vi "get raw data.vi"(8 "error in (no error)":errorcluster, 11 "Task.lvclass in":refnum<class "Task.lvclass">) -> (0 "error out":errorcluster, 2 "data":T1, 3 "Task.lvclass out":refnum<class "Task.lvclass">)   [LabVIEW 2020, in "Tasks.lvlib" / "Task.lvclass"]
uses:
  Task.lvclass
  data.ctl
  SignalConversion/DAQChannelRawData.ctl
  Task.lvclass/Task.ctl
  SignalConversion/SignalConverson.lvlib
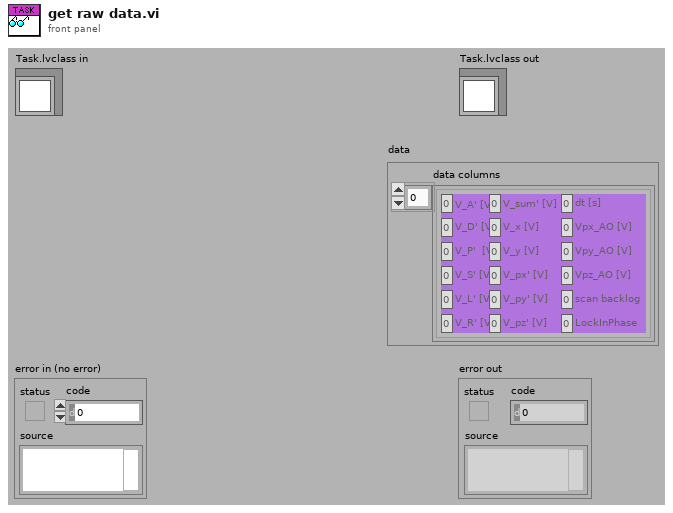
[diagram p1: front panel]
types:
  T1 = typedef "Tasks.lvlib/Task.lvclass/data.ctl" = cluster{"data columns":T2[]}
  T2 = typedef "SignalConverson.lvlib/DAQChannelRawData.ctl" = cluster{"V_A' [V]":dbl, "V_D' [V]":dbl, "V_P'  [V]":dbl, "V_S' [V]":dbl, "V_L' [V]":dbl, "V_R' [V]":dbl, "V_sum' [V]":dbl, "V_x [V]":dbl, "V_y [V]":dbl, "V_px' [V]":dbl, "V_py' [V]":dbl, "V_pz' [V]":dbl, "dt [s]":dbl, "Vpx_AO [V]":dbl, "Vpy_AO [V]":dbl, "Vpz_AO [V]":dbl, "scan backlog":u32, "LockInPhase":dbl}
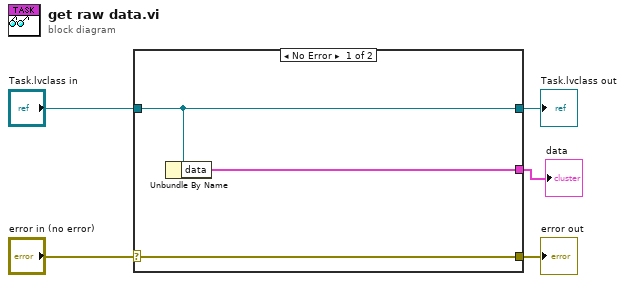
[diagram p0: block diagram]
diagram:
  n1 = case shown="No Error" "error in (no error)" {
    selector: "error in (no error)" -> [w8 w9]
    tunnel: [w8 w9] -> w4
    tunnel: [w7 w10] -> w2
    tunnel: "Task.lvclass in" -> [w7 w10]
    tunnel: [w6 _] -> w1
    frame No Error {
      n2 = Unbundle By Name(w7) -> ("data"=w6:T1)
    }
    frame Error {
    }
  }
  "error out" <- w4
  "Task.lvclass out" <- w2
  "data" <- w1
